vi "DisableOutput.vi"(8 "Error In":errorcluster, 11 "Keithley 6482 In":refnum<visa-resource-name>) -> (0 "Error Out":errorcluster, 3 "Keithley 6482 Out":refnum<visa-resource-name>)   [LabVIEW 2010, in "Keithley-6482-Visa.lvlib"]
uses:
  <instrlib>/lib-labview-8.6-export/Keithley-6482-Visa.lvlib
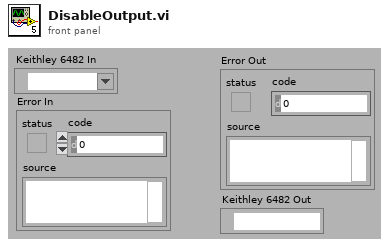
[diagram p1: front panel]
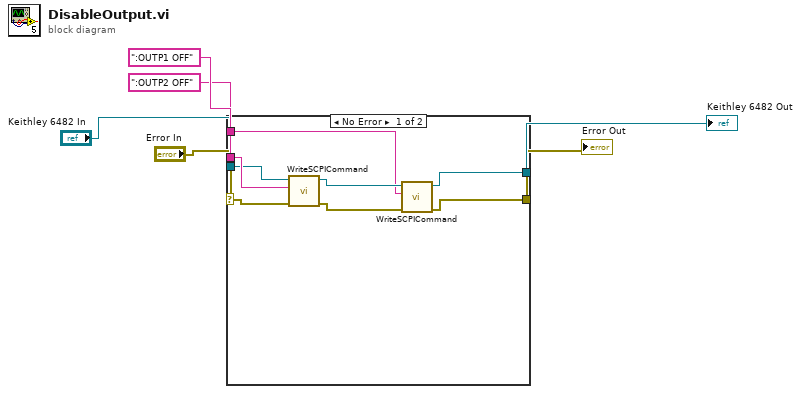
[diagram p0: block diagram]
diagram:
  n1 = case shown="No Error" "Error In" {
    selector: "Error In" -> [w12 w15]
    tunnel: ":OUTP1 OFF" -> [w14 _]
    tunnel: "Keithley 6482 In" -> [w13 w16]
    tunnel: [w10 w16] -> w3
    tunnel: [w8 w15] -> w2
    tunnel: ":OUTP2 OFF" -> [w7 _]
    frame No Error {
      n2 = call <instrlib>:"WriteSCPICommand.vi"("Error In"=w12, "SCPI Command"=w14, "Keithley 6482 In"=w13) -> ("Error Out"=w9:errorcluster, "Keithley 6482 Out"=w11:refnum<visa-resource-name>)  [unwired: 7 in]
      n3 = call <instrlib>:"WriteSCPICommand.vi"("Error In"=w9, "SCPI Command"=w7, "Keithley 6482 In"=w11) -> ("Error Out"=w8:errorcluster, "Keithley 6482 Out"=w10:refnum<visa-resource-name>)  [unwired: 7 in]
    }
    frame Error {
    }
  }
  "Error Out" <- w2
  "Keithley 6482 Out" <- w3
